vi "Simulador CLP.vi"(8 "String lido da placa":string, 11 "String vindo do OPC":string) -> (0 "String para OPC":string, 3 "String para Placa Freescale":string)   [LabVIEW 2019]
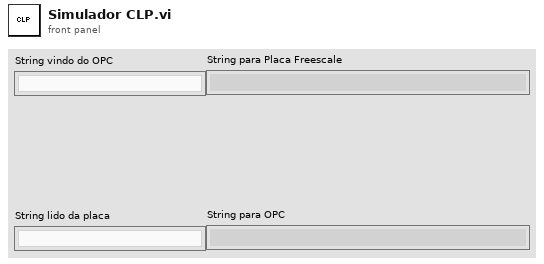
[diagram p1: front panel]
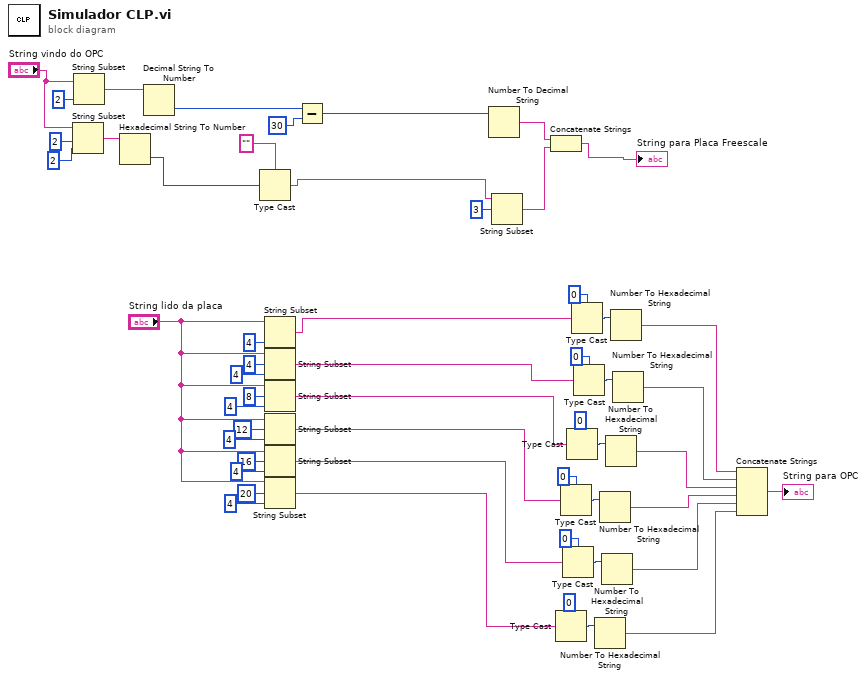
[diagram p0: block diagram]
diagram:
  n1 = String Subset(string="String vindo do OPC", offset (0)=2, length (rest)=2 ("length (rest)")) -> (substring=w6:string)
  n2 = String Subset(string="String vindo do OPC", length (rest)=2 ("length (rest)")) -> (substring=w49:string)  [unwired: 1 in]
  n3 = Hexadecimal String To Number(string=w6) -> (number=w4:u32)  [unwired: 2 in, 1 out]
  n4 = Decimal String To Number(string=w49) -> (number=w48:i32)  [unwired: 2 in, 1 out]
  n5 = Type Cast(type="", x=w4) -> (*(type *) &x=w2:string)
  n6 = String Subset(string="String lido da placa", length (rest)=4 ("length (rest)")) -> (substring=w44:string)  [unwired: 1 in]
  n7 = String Subset(string="String lido da placa", offset (0)=4, length (rest)=4 ("length (rest)")) -> (substring=w36:string)
  n8 = String Subset(string="String lido da placa", offset (0)=8, length (rest)=4 ("length (rest)")) -> (substring=w33:string)
  n9 = String Subset(string="String lido da placa", offset (0)=12, length (rest)=4 ("length (rest)")) -> (substring=w20:string)
  n10 = String Subset(string="String lido da placa", offset (0)=16, length (rest)=4 ("length (rest)")) -> (substring=w19:string)
  n11 = String Subset(string="String lido da placa", offset (0)=20, length (rest)=4 ("length (rest)")) -> (substring=w18:string)
  n12 = Subtract(x=w48, y=30) -> (x-y=w9:i32)
  n13 = Number To Decimal String(number=w9) -> (decimal integer string=w7:string)  [unwired: 1 in]
  n14 = String Subset(string=w2, offset (0)=3) -> (substring=w1:string)  [unwired: 1 in]
  n15 = Concatenate Strings(w7, w1) -> (→"String para Placa Freescale":string)
  n16 = Type Cast(type=0, x=w18) -> (*(type *) &x=w21:i32)
  n17 = Type Cast(type=0, x=w20) -> (*(type *) &x=w25:i32)
  n18 = Type Cast(type=0, x=w19) -> (*(type *) &x=w23:i32)
  n19 = Type Cast(type=0, x=w33) -> (*(type *) &x=w34:i32)
  n20 = Type Cast(type=0, x=w44) -> (*(type *) &x=w45:i32)
  n21 = Type Cast(type=0, x=w36) -> (*(type *) &x=w37:i32)
  n22 = Number To Hexadecimal String(2:w21) -> (0:w11:string)  [unwired: 1 in]
  n23 = Number To Hexadecimal String(2:w25) -> (0:w13:string)  [unwired: 1 in]
  n24 = Number To Hexadecimal String(2:w23) -> (0:w12:string)  [unwired: 1 in]
  n25 = Number To Hexadecimal String(2:w34) -> (0:w14:string)  [unwired: 1 in]
  n26 = Number To Hexadecimal String(2:w45) -> (0:w16:string)  [unwired: 1 in]
  n27 = Number To Hexadecimal String(2:w37) -> (0:w15:string)  [unwired: 1 in]
  n28 = Concatenate Strings(w16, w15, w14, w13, w12, w11) -> (→"String para OPC":string)
